vi "Create.vi"(5 "TestCaseMock In":refnum<class "TestCaseMock.lvclass">, 8 "error in (no error)":errorcluster) -> (0 "error out":errorcluster, 3 "TestCaseMock":refnum<class "TestCaseMock.lvclass">)   [LabVIEW 2019, in "TestResultTestSupport.lvlib" / "TestCaseMock.lvclass"]
uses:
  TestCaseMock.lvclass
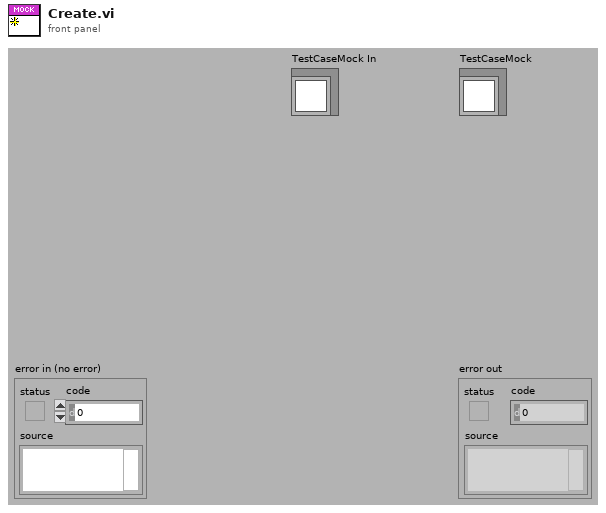
[diagram p1: front panel]
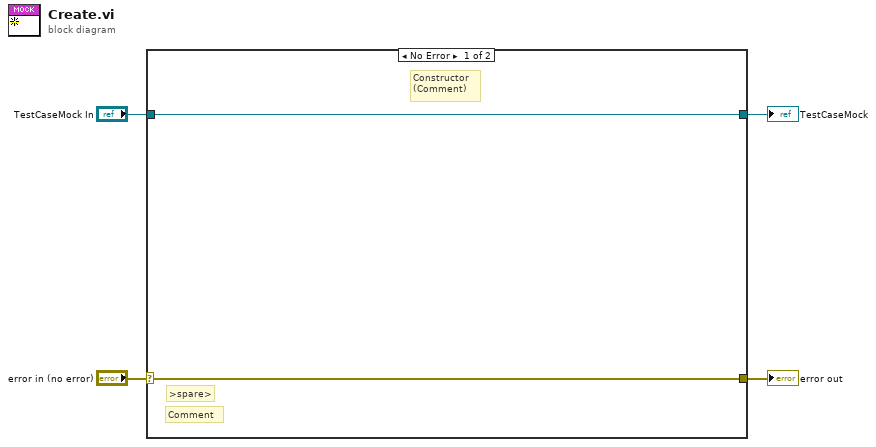
[diagram p0: block diagram]
diagram:
  n1 = case shown="No Error" "error in (no error)" {
    selector: "error in (no error)" -> [w6 w8]
    tunnel: [w6 w8] -> w3
    tunnel: [w5 w7] -> w1
    tunnel: "TestCaseMock In" -> [w5 w7]
    frame No Error {
      # ">spare>"
      # "Constructor\n(Comment)"
      # "Comment"
    }
    frame Error {
    }
  }
  "error out" <- w3
  "TestCaseMock" <- w1
